vi "2048_generate_new_element.vi"(11 "Array in":i32[][](array[numeric])) -> (0 "c":u64, 1 "r":u64, 2 "element":i16, 3 "Array out":i32[][](array[numeric]))   [LabVIEW 2022 SP3]
uses:
  <vilib>/numeric/Random Number (Range) U64.vi
  <vilib>/numeric/Random Number (Range) I64.vi
  <vilib>/numeric/sub_Random U32.vi
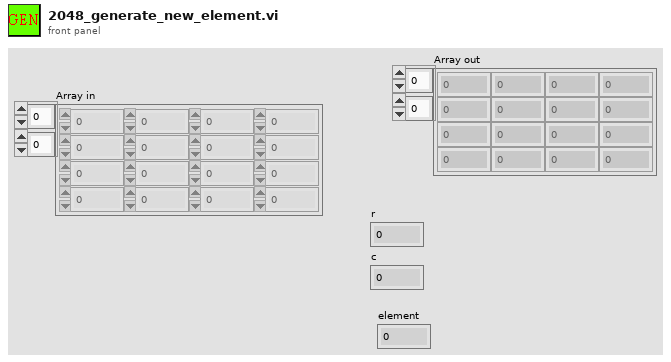
[diagram p1: front panel]
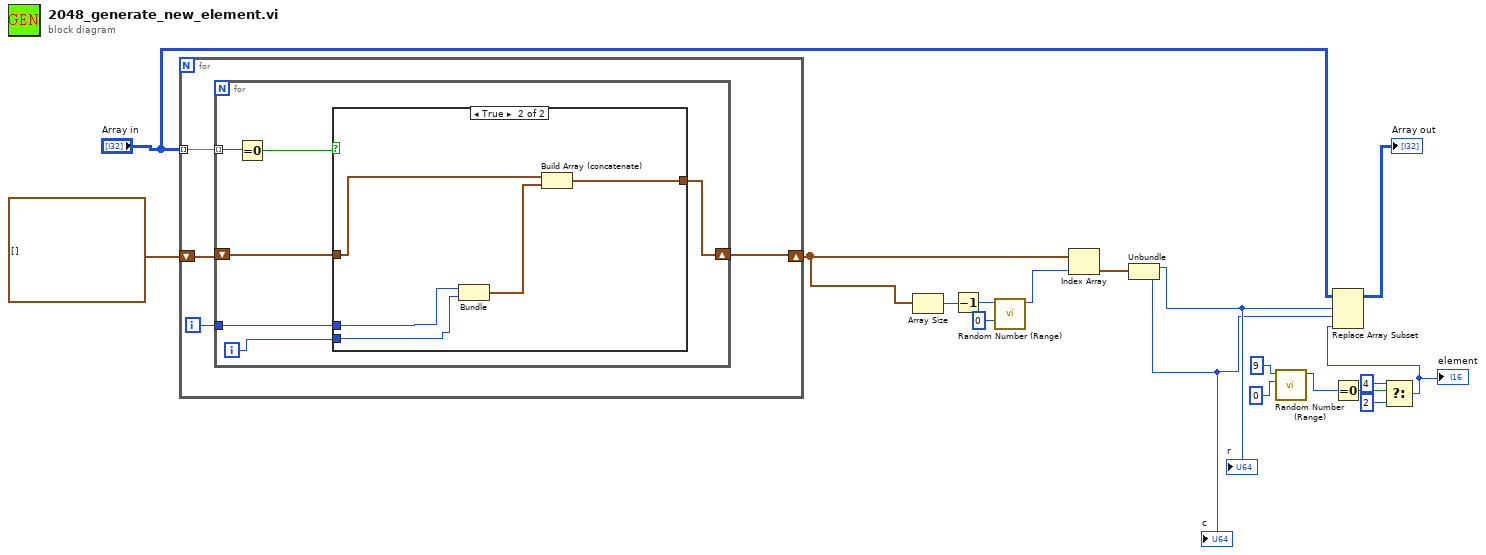
[diagram p0: block diagram]
diagram:
  n1 = for {
    tunnel: "Array in" -> [w22] mode=indexing
    shift-right: [w19] -> w5
    shift-left: cluster{i32, i32}[] [] -> [w21]
    i -> [w20]
    n2 = for {
      tunnel: w22 -> [w28] mode=indexing
      shift-right: [w23] -> w19
      shift-left: w21 -> [w26]
      tunnel: w20 -> [w25]
      i -> [w24]
      n3 = Equal To 0?(x=w28) -> (x = 0?=w27:bool)
      n4 = case shown="True" w27 {
        tunnel: w26 -> [w29 w34]
        tunnel: w25 -> [_ w32]
        tunnel: w24 -> [_ w31]
        tunnel: [w29 w33] -> w23
        frame False {
        }
        frame True {
          n5 = Bundle(w32, w31) -> (w30:cluster{i32, i32})  [unwired: 1 in]
          n6 = Build Array (concatenate)(w34, w30) -> (w33:cluster{i32, i32}[])
        }
      }
    }
  }
  n7 = Array Size(array=w5) -> (size(s)=w9:i32)
  n8 = Decrement(x=w9) -> (x-1=w8:i32)
  n9 = call-poly <vilib>:"Random Number (Range).vi"("lower bound (-100)"=i64 0, "upper bound (100)"=w8) -> ("number"=w6:i64)  [unwired: 9 in]
  n10 = Index Array(array=w5, index=w6) -> (element=w4:cluster{i32, i32})
  n11 = Unbundle(w4) -> (w3:i32, w2:i32)
  "r" <- w3
  "c" <- w2
  n12 = call-poly <vilib>:"Random Number (Range).vi"("lower bound (0)"=u64 0, "upper bound (100)"=u64 9) -> ("number"=w15:u64)  [unwired: 9 in]
  n13 = Equal To 0?(x=w15) -> (x = 0?=w14:bool)
  n14 = Select(t=i16 4, s=w14, f=i16 2) -> (s? t:f=w11:i16)
  "element" <- w11
  n15 = Replace Array Subset(array="Array in", new element=w11, index (row)=w3, index (col)=w2) -> (→"Array out":i32[][])
